vi "Read Worker-Object Name.vi"(8 "error in (no error)":errorcluster, 11 "CS++PVProxy in":refnum<class "CS++PVProxy.lvclass">) -> (0 "error out":errorcluster, 2 "Worker-Object Name":string, 3 "CS++PVProxy out":refnum<class "CS++PVProxy.lvclass">)   [LabVIEW 2015, in "CS++PVProxy.lvlib" / "CS++PVProxy.lvclass"]
doc: "Read name of worker actor."
uses:
  CS++PVProxy.lvclass
  CS++PVProxy.lvclass/CS++PVProxy.ctl
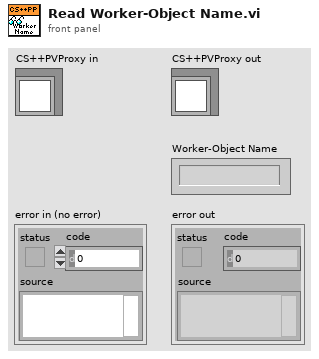
[diagram p1: front panel]
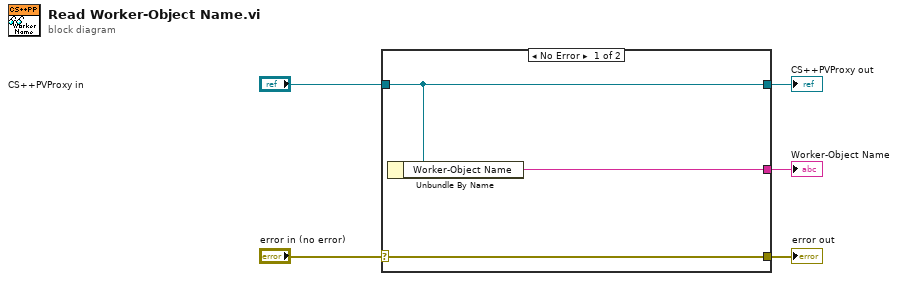
[diagram p0: block diagram]
diagram:
  n1 = case shown="No Error" "error in (no error)" {
    selector: "error in (no error)" -> [w8 w9]
    tunnel: [w8 w9] -> w4
    tunnel: [w7 w10] -> w2
    tunnel: "CS++PVProxy in" -> [w7 w10]
    tunnel: [w6 _] -> w1
    frame No Error {
      n2 = Unbundle By Name(w7) -> ("Worker-Object Name"=w6:string)
    }
    frame Error {
    }
  }
  "error out" <- w4
  "CS++PVProxy out" <- w2
  "Worker-Object Name" <- w1
